vi "SetGenNOscL0MAJMan.vi"(5 "Input Voltage":dbl=0.2, 6 "Amp Scaler":dbl=1.0, 7 "NChannels":i32, 8 "error in (no error)":errorcluster, 9 "Output Voltage":dbl=0.2, 10 "VISA resource name":refnum<visa-resource-name>="AgilentOsciloscope", 11 "AWG VISA":refnum<visa-resource-name>="AgilentGenerator1") -> (0 "error out 2":errorcluster={"status"=TRUE, "code"=-1074000000, "source"="Agilent 8000 Series.lvlib:Error Query.vi<ERR>\nInstrument reports:\n-222,\"Data out of range\"\r\n0,\"No error\"\r\n\n\n\n<b>Complete call chain:</b>\r\n     Agilent 8000 Series.lvlib:Error Query.vi\r\n     Agilent 8000 Series.lvlib:Configure Channel.vi\r\n     SetGenNOscL0MAJMan.vi"})   [LabVIEW 2012]
uses:
  <instrlib>/Agilent 8000 Series/Agilent 8000 Series.lvlib
  Sum_Abrilader/L0_Sum_Adder Folder/C/Program Files/National Instruments/LabVIEW 2012/instr.lib/Agilent 81150/Agilent 81150.lvlib
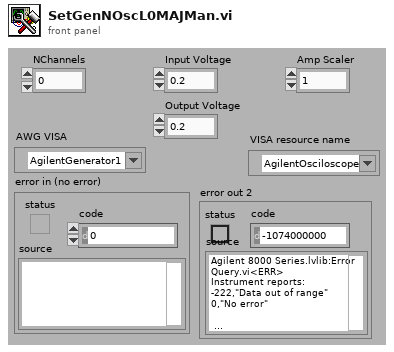
[diagram p1: front panel]
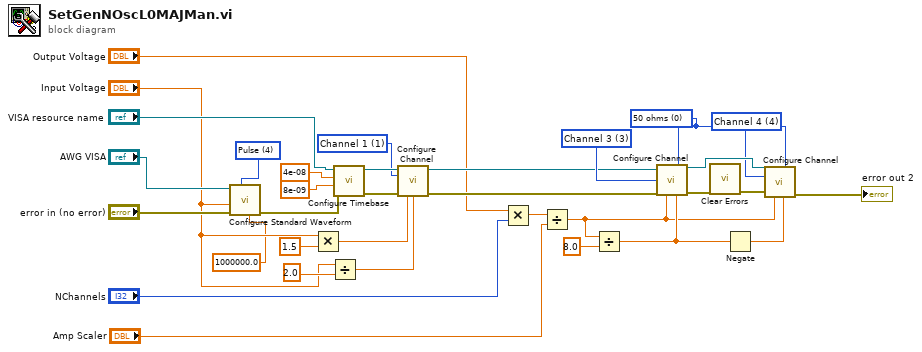
[diagram p0: block diagram]
diagram:
  w21 = u32 0 items=["50 ohms", "1 Mohms"] ("Input Impedance (1: 1 Mohms)")
  w19 = 3 items=["Channel 1"=1, "Channel 2"=2, "Channel 3"=3, "Channel 4"=4] ("Channel (1: Channel 1)")
  w18 = 4 items=["Channel 1"=1, "Channel 2"=2, "Channel 3"=3, "Channel 4"=4] ("Channel (1: Channel 1)")
  w25 = 1 items=["Channel 1"=1, "Channel 2"=2, "Channel 3"=3, "Channel 4"=4] ("Channel (1: Channel 1)")
  w4 = u16 4 items=["Sine", "Square", "Ramp Up", "Ramp Down", "Pulse", "Noise", "DC"] ("Waveform (0: Sine)")
  n1 = call <instrlib>:"Configure Standard Waveform.vi"("Frequency (1000.0 Hz)"=1000000.0, "Waveform (0: Sine)"=w4, "error in (no error)"="error in (no error)", "Amplitude (1.0 Vpp)"="Input Voltage", "VISA resource name"="AWG VISA") -> ("error out"=w5:errorcluster)  [unwired: 5 in, 1 out]
  n2 = Multiply(x="Input Voltage", y=1.5) -> (x*y=w29:dbl)
  n3 = Divide(x="Input Voltage", y=2.0) -> (x/y=w26:dbl)
  n4 = call "Configure Timebase.vi"("error in (no error)"=w5, "Position (0.0 s)"=8e-09, "Timebase (0.005 s)"=4e-08, "VISA resource name"="VISA resource name") -> ("error out"=w33:errorcluster, "VISA resource name out"=w32:refnum<visa-resource-name>)  [unwired: 6 in]
  n5 = call <instrlib>:"Configure Channel.vi"("VISA resource name"=w32, "Channel (1: Channel 1)"=w25, "error in (no error)"=w33, "Vertical Range (2.0 V)"=w29, "Vertical Offset (0.0 V)"=w26) -> ("VISA resource name out"=w13:refnum<visa-resource-name>, "error out"=w12:errorcluster)  [unwired: 9 in]
  n6 = Multiply(x="Output Voltage", y="NChannels") -> (x*y=w14:dbl)
  n7 = Divide(x=w14, y="Amp Scaler") -> (x/y=w9:dbl)
  n8 = Divide(x=w9, y=8.0) -> (x/y=w15:dbl)
  n9 = call <instrlib>:"Configure Channel.vi"("VISA resource name"=w13, "Input Impedance (1: 1 Mohms)"=w21, "Channel (1: Channel 1)"=w19, "error in (no error)"=w12, "Vertical Range (2.0 V)"=w9, "Vertical Offset (0.0 V)"=w15) -> ("VISA resource name out"=w22:refnum<visa-resource-name>, "error out"=w23:errorcluster)  [unwired: 8 in]
  n10 = call <vilib>:"Clear Errors.vi"("error in (no error)"=w23) -> ("error out"=w20:errorcluster)  [unwired: 6 in]
  n11 = Negate(x=w15) -> (-x=w17:dbl)
  n12 = call <instrlib>:"Configure Channel.vi"("VISA resource name"=w22, "Input Impedance (1: 1 Mohms)"=w21, "Channel (1: Channel 1)"=w18, "error in (no error)"=w20, "Vertical Range (2.0 V)"=w9, "Vertical Offset (0.0 V)"=w17) -> ("error out"=→"error out 2":errorcluster)  [unwired: 8 in, 1 out]
